vi "VFD Control Loop.vi"(8 "error in (no error)":errorcluster, 10 "VFD Notifier":refnum<notifier>, 11 "Message Queues":T2) -> (0 "error out":errorcluster)   [LabVIEW 2026]
uses:
  support/Message Queue/All Message Queues.ctl
  support/Message Queue/Message Cluster.ctl
  controls/VFD Notifier ctl.ctl
  Acquisition/Hardware Configuration.ctl
  controls/Durability Test Conditions.ctl
  Acquisition/Acquisition State.ctl
  VFD-Library-main/VFD-Library-main/Public/Action/Direction Selection.ctl
  support/Message Queue/Enqueue Message (Single).vi
  <vilib>/Utility/error.llb/Error Cluster From Error Code.vi
  <vilib>/ErrorRing/Error Ring.xnode
  Acquisition/Acquisition.lvlib
  support/Message Queue/Message Queue.lvlib
  VFD-Library-main/VFD-Library-main/VFD Library.lvlib
panel:
  in  "Cluster":T1={"Voltage"=0.0, "Current"=0.0, "Motor Speed"=0.0, "Fault"=TRUE, "Fault Messages"=[]}
  out "Faults":string[](array[string])
  out "Fault":bool
  out "Motor feedback\nspeed":dbl format="%#_13g"
  out "Current":dbl format="%#_13g"
  out "Voltage":dbl format="%#_13g"
  in  "IP Address":string="172.20.0.115"
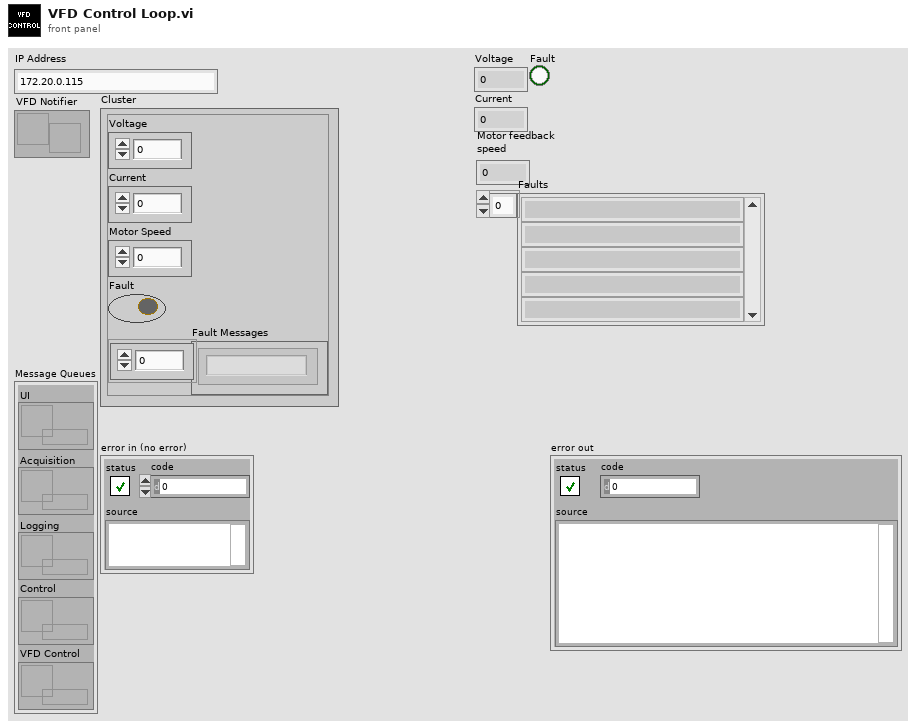
[diagram p1: front panel]
types:
  T1 = typedef "VFD Notifier ctl.ctl" = cluster{"Voltage":dbl, "Current":dbl, "Motor Speed":dbl, "Fault":bool, "Fault Messages":string[]}
  T2 = typedef "Message Queue.lvlib/All Message Queues.ctl" = cluster{"UI":refnum<queue>, "Acquisition":refnum<queue>, "Logging":refnum<queue>, "Control":refnum<queue>, "VFD Control":refnum<queue>}
  T3 = typedef "Acquisition.lvlib/Hardware Configuration.ctl" = cluster{"Analog Out array":dbl[], "Initialize Flag":bool, "Saftey Table Display":refnum<vi>, "Torque&Force":waveform(dbl)[][], "Calibration Data":waveform(dbl)[], "2D":dbl[][], "Analog In Task":refnum<k21>, "Digital In Task":refnum<k21>, "Analog Out Task":refnum<k21>, "Digital Out Task":refnum<k21>, "Digital Out Array":bool[], "Current Cycle Count":refnum<vi>, "Cycle Count":u64, "Headers":string[], "Sweep Interval":u64, "Delay":u64, "TestConfigDisplay":refnum<vi>, "50psi Conversion":dbl[], "1245N15 Conversion":dbl[], "MX06F Conversion":dbl[], "# of Test Cycles":u64, "60psi Conversion":dbl[], "100psi Conversion":dbl[], "200psi Conversion":dbl[], "1000psi Conversion":dbl[], "2000psi Conversion":dbl[], "5000psi Conversion":dbl[], "MX09F Conversion":dbl[], "MX19F Conversion":dbl[], "DUT VALVE POSITION":refnum<vi>, "INTAKE VALVE POSITION":refnum<vi>, "Table Control":refnum<vi>, "Table Control":string[][], "Max Vacuum":dbl, "RPM Ramp Ref":refnum<vi>, "Free Air Flow Ref":refnum<vi>, "Press Stable Ref":refnum<vi>, "Press Decay Ref":refnum<vi>, "Pulley Ratio":dbl, "Calculated Pulley Ratio":refnum<vi>, "Durability Test Conditions":T4, "# of Durab Steps":dbl, "manual aquire timer":dbl, "Durability Test Conditions Initial":T4}
  T4 = typedef "Durability Test Conditions.ctl" = cluster{"Step #s":dbl[], "RPMs":dbl[], "Step Durations":dbl[], "Step Delays":dbl[], "Test Cycles":dbl}
  T5 = typedef "Acquisition.lvlib/Acquisition State.ctl" = enum16{"Idle", "Acquiring"}
  T6 = typedef "VFD Library.lvlib/Direction Selection.ctl" = u16
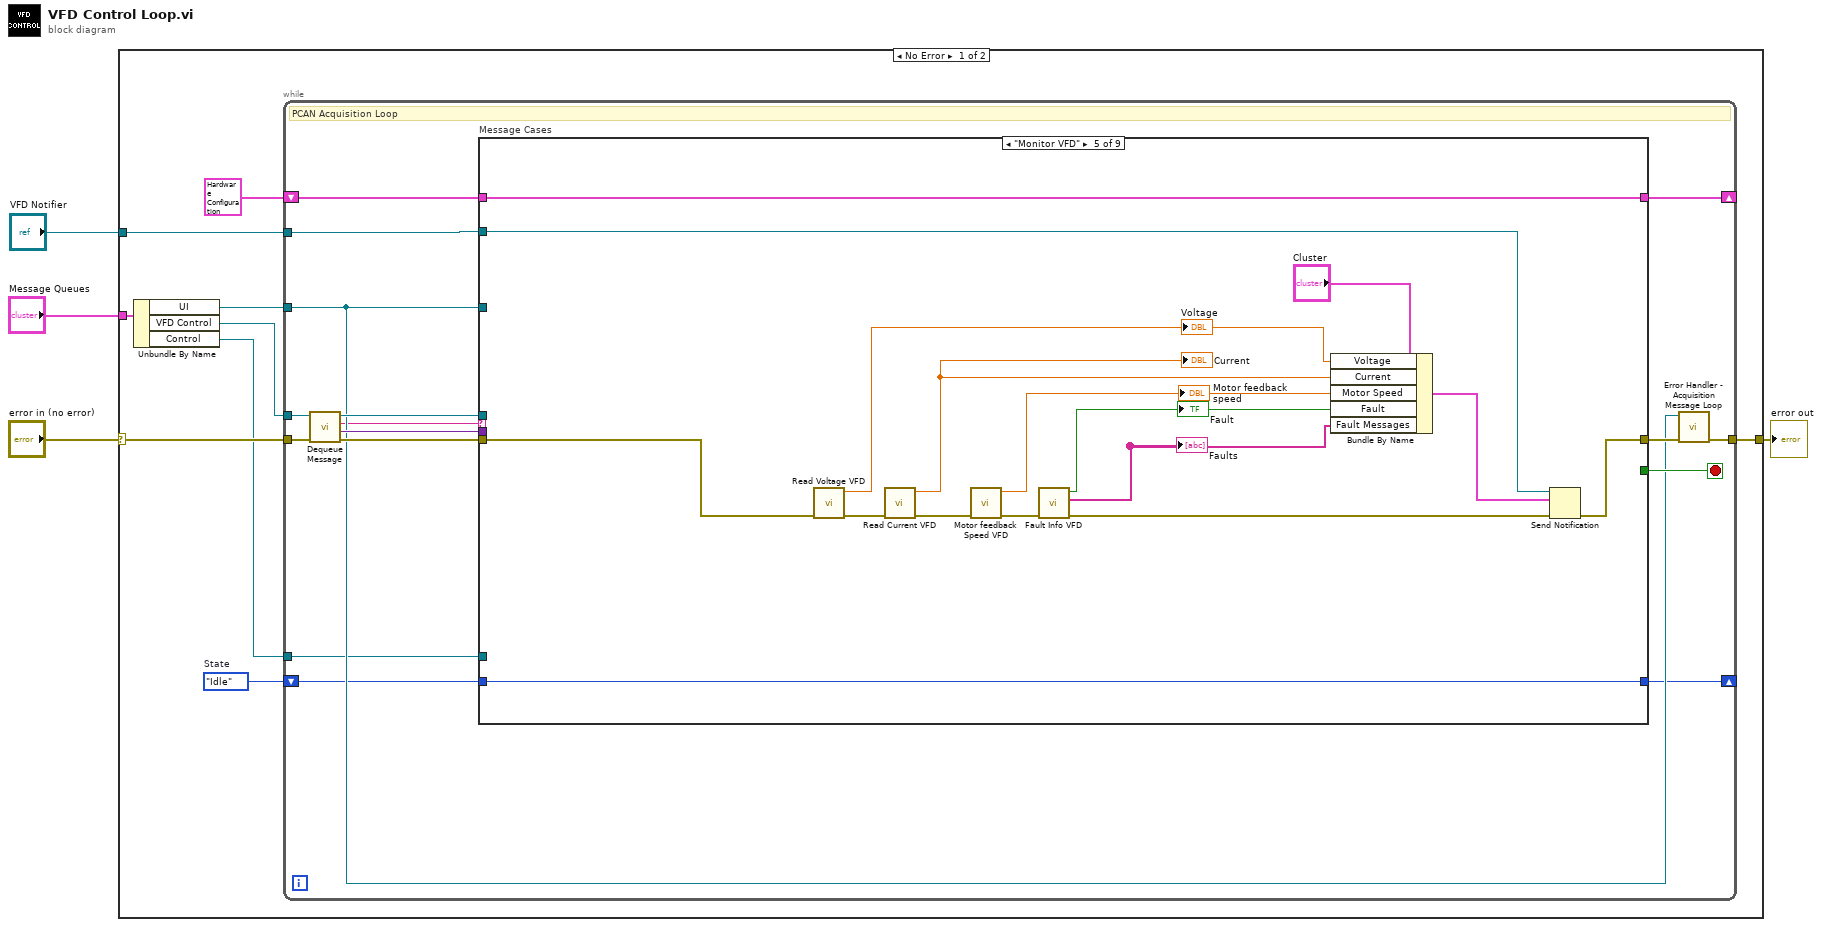
[diagram p0: block diagram]
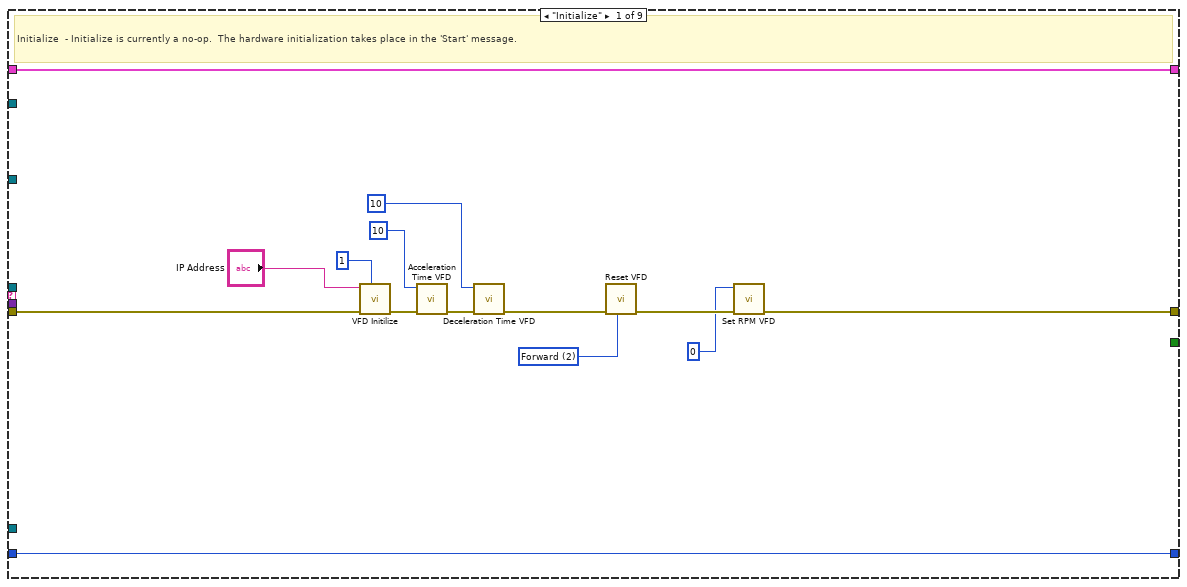
[diagram p2: hidden frame]
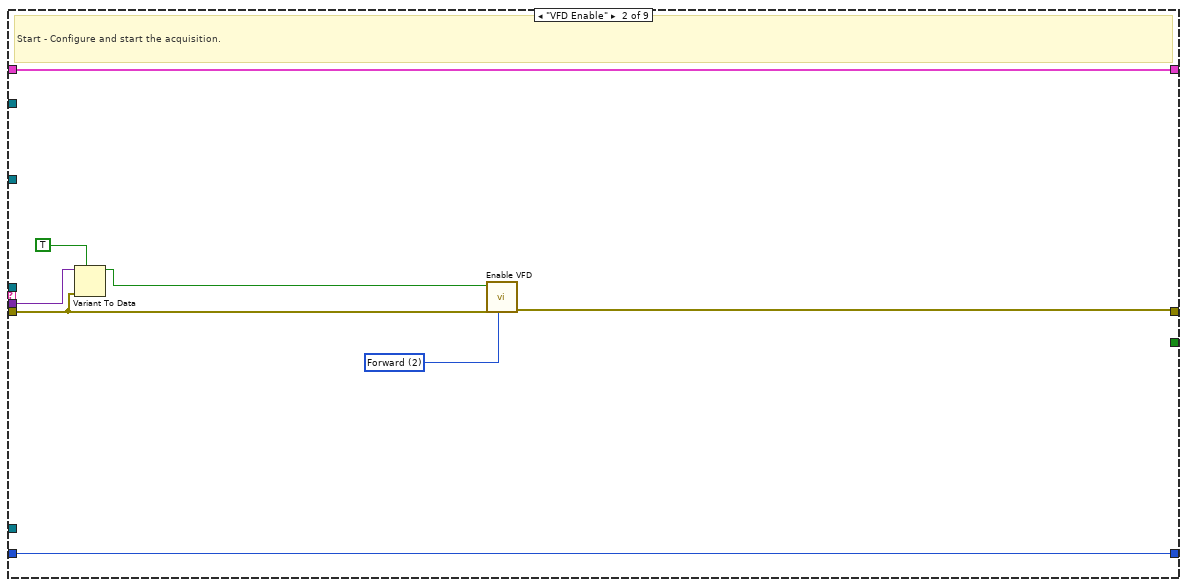
[diagram p3: hidden frame]
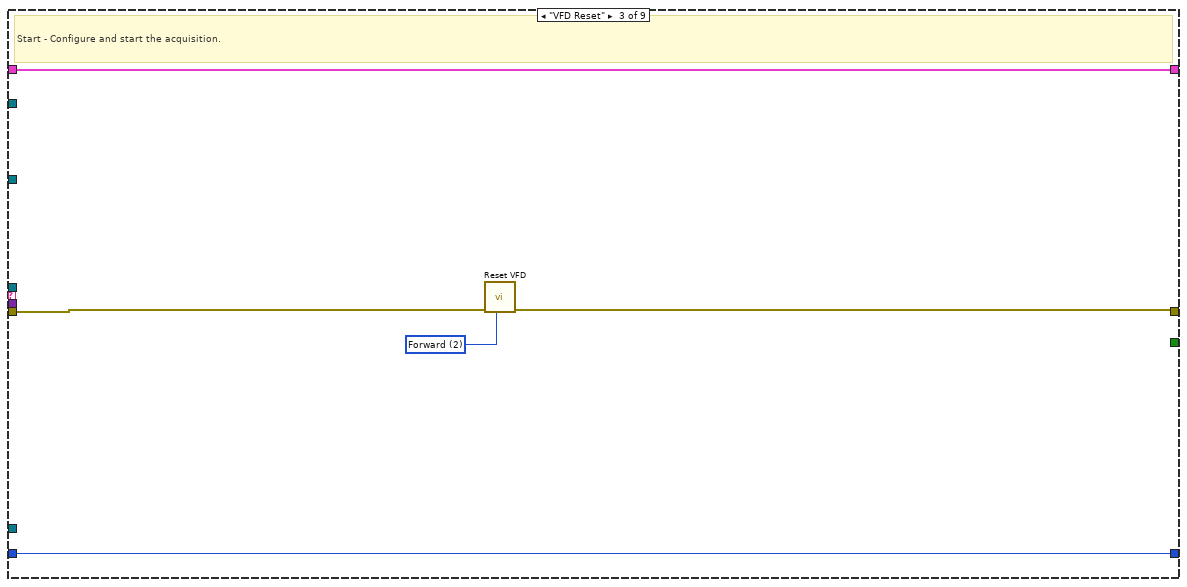
[diagram p4: hidden frame]
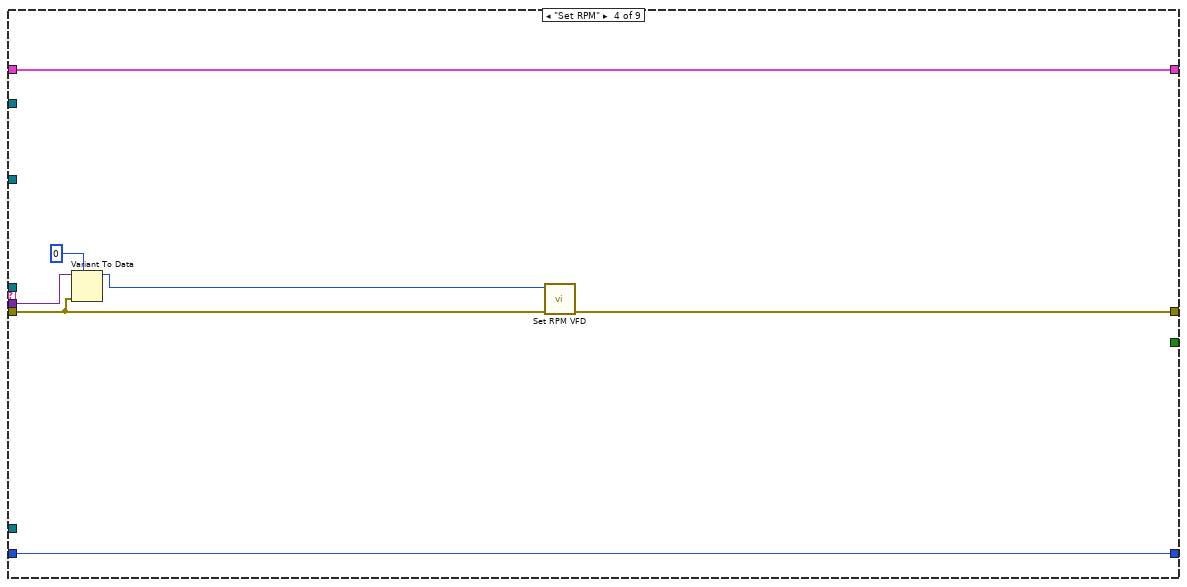
[diagram p5: hidden frame]
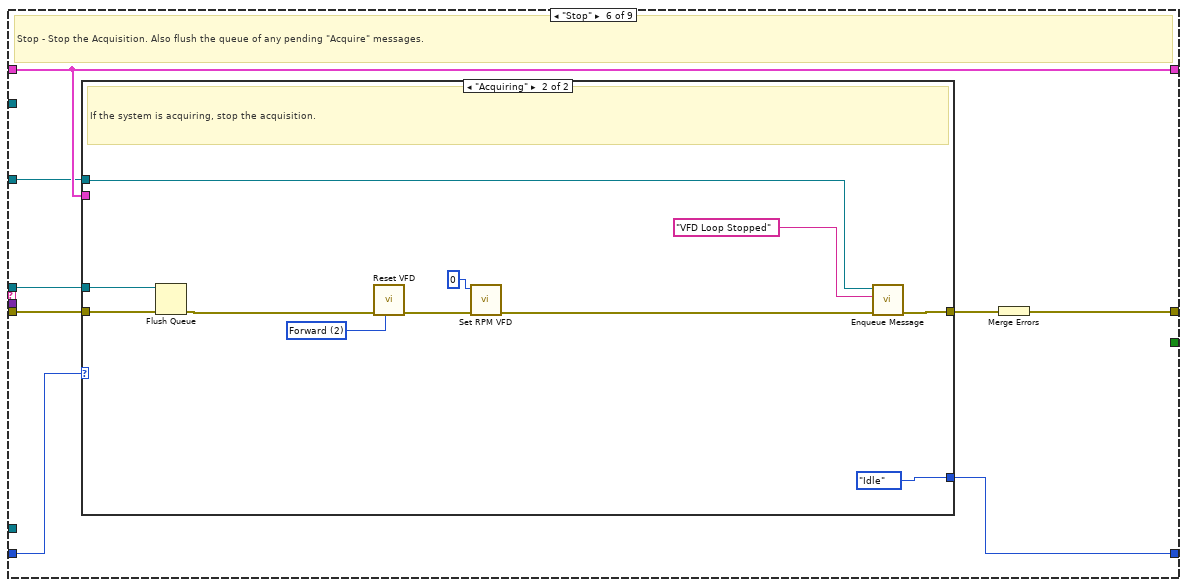
[diagram p6: hidden frame]
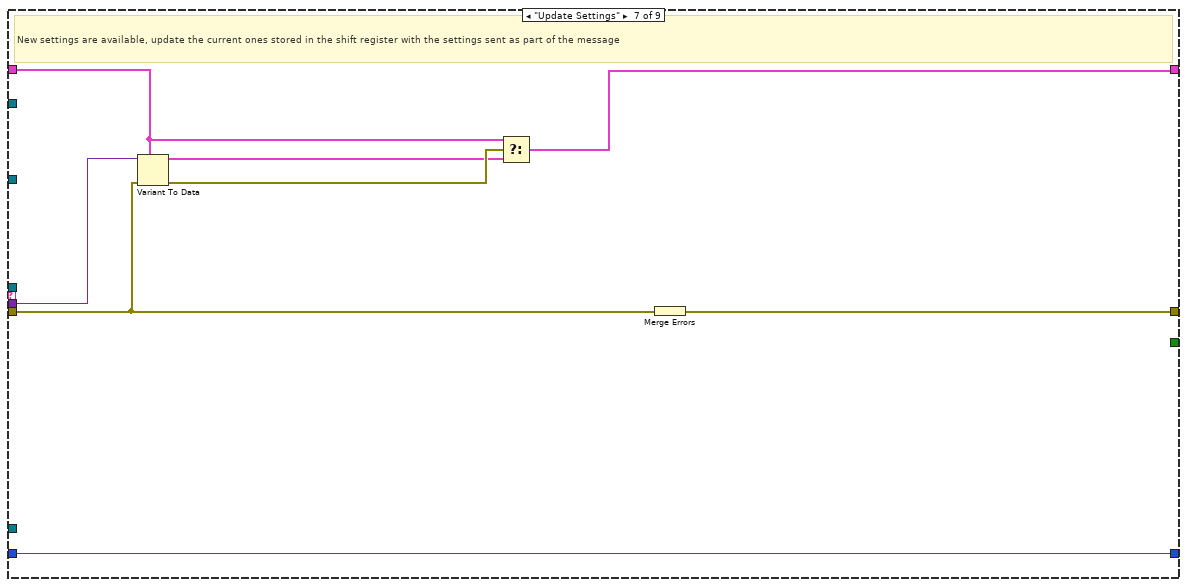
[diagram p8: hidden frame]
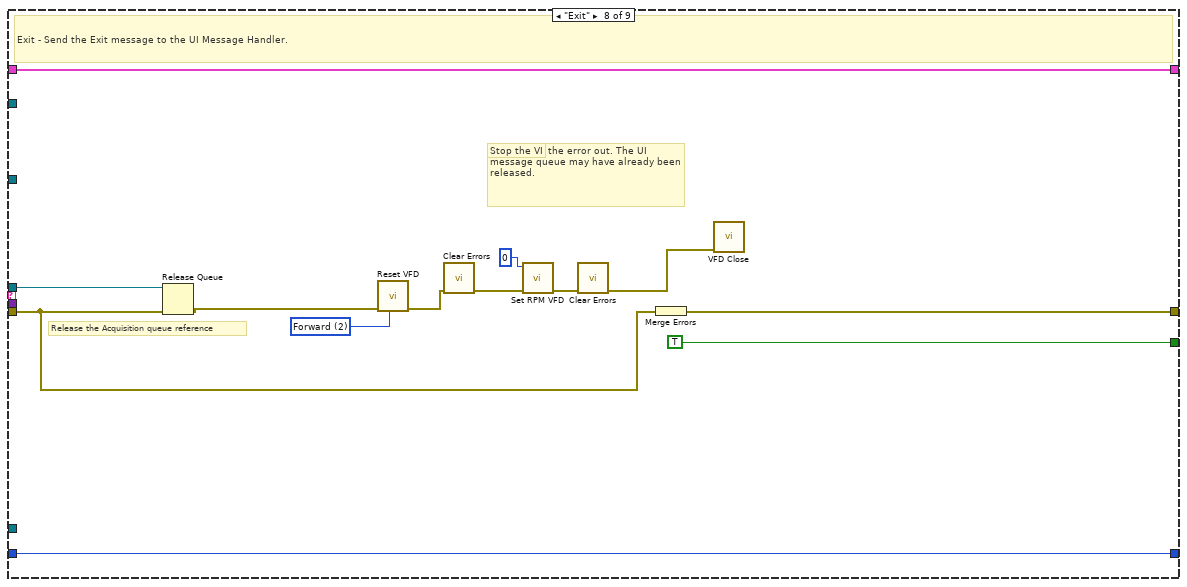
[diagram p9: hidden frame]
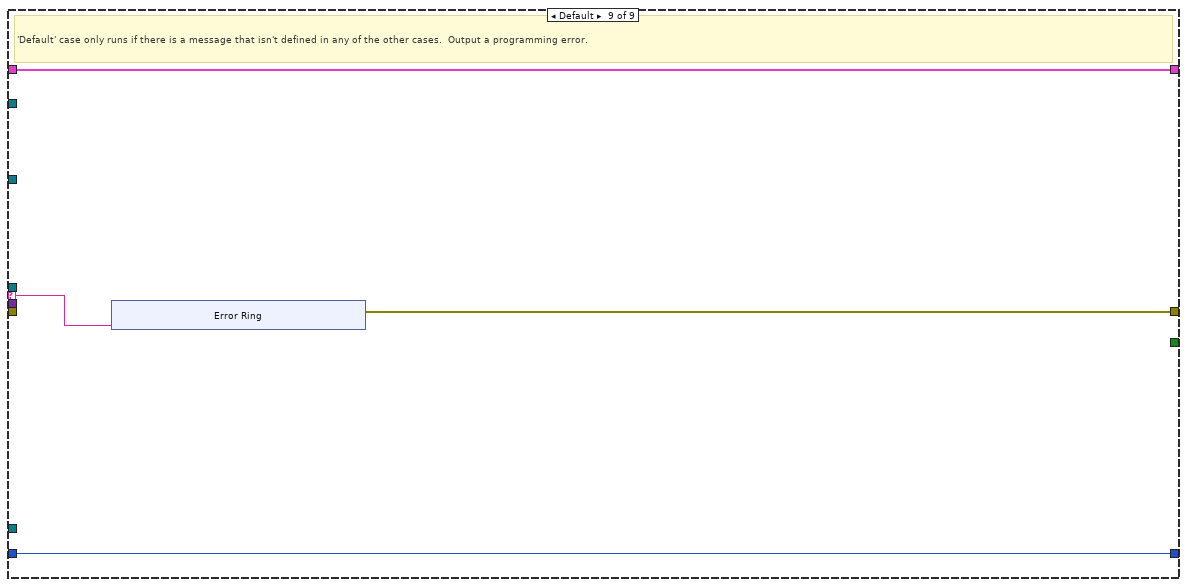
[diagram p10: hidden frame]
diagram:
  n1 = case shown="No Error" "error in (no error)" {
    selector: "error in (no error)" -> [w10 w133]
    tunnel: "Message Queues" -> [w13 _]
    tunnel: [w12 w133] -> w3
    tunnel: "VFD Notifier" -> [w5 _]
    frame No Error {
      w8 = Acquisition_State."Idle"  # State
      n2 = Unbundle By Name(w13) -> ("UI"=w9:refnum<queue>, "VFD Control"=w6:refnum<queue>, "Control"=w7:refnum<queue>)
      n3 = while {
        tunnel: w6 -> [w22]
        shift-right: [w28] -> _
        shift-left: T3 {"Analog Out array"=[], "Initialize Flag"=FALSE, "Saftey Table Display"=refnum, "Torque&Force"=[], "Calibration Data"=[], "2D"=[], "Analog In Task"="", "Digital In Task"="", "Analog Out Task"="", "Digital Out Task"="", "Digital Out Array"=[], "Current Cycle Count"=refnum, "Cycle Count"=0, "Headers"=[], "Sweep Interval"=0, "Delay"=0, "TestConfigDisplay"=refnum, "50psi Conversion"=[], "1245N15 Conversion"=[], "MX06F Conversion"=[], "# of Test Cycles"=0, "60psi Conversion"=[], "100psi Conversion"=[], "200psi Conversion"=[], "1000psi Conversion"=[], "2000psi Conversion"=[], "5000psi Conversion"=[], "MX09F Conversion"=[], "MX19F Conversion"=[], "DUT VALVE POSITION"=refnum, "INTAKE VALVE POSITION"=refnum, "Table Control"=refnum, "Table Control"=[], "Max Vacuum"=0.0, "RPM Ramp Ref"=refnum, "Free Air Flow Ref"=refnum, "Press Stable Ref"=refnum, "Press Decay Ref"=refnum, "Pulley Ratio"=0.0, "Calculated Pulley Ratio"=refnum, "Durability Test Conditions"={"Step #s"=[], "RPMs"=[], "Step Durations"=[], "Step Delays"=[], "Test Cycles"=0.0}, "# of Durab Steps"=0.0, "manual aquire timer"=0.0, "Durability Test Conditions Initial"={"Step #s"=[], "RPMs"=[], "Step Durations"=[], "Step Delays"=[], "Test Cycles"=0.0}} ("Data Cluster") -> [w29]
        tunnel: w9 -> [w19]
        shift-right: [w17] -> _
        shift-left: w8 -> [w18]
        tunnel: w7 -> [w16]
        tunnel: w10 -> [w26]
        tunnel: [w20] -> w12
        tunnel: w5 -> [w15]
        stop <- w27 stop-if-true
        # "PCAN Acquisition Loop"
        n4 = call "Dequeue Message.vi"("error in (no error)"=w26, "Message Queue"=w22) -> ("error out"=w25:errorcluster, "Message Data"=w24:variant, "Message"=w14:string, "dup Message Queue"=w23:refnum<queue>)  [unwired: 6 in]
        n5 = case "Message Cases" shown="\"Monitor VFD\"" w14 {
          selector: w14 -> [_ _ _ _ _ _ _ _ w124]
          tunnel: w23 -> [_ _ _ _ _ w84 _ w119 _]
          tunnel: w25 -> [w35 w47 w54 w60 w75 w86 w102 w116 _]
          tunnel: [w32 w49 w53 w61 w72 w87 w108 w120 w123] -> w21
          tunnel: w29 -> [w42 w50 w55 w62 w79 w85 w104 w117 w125]
          tunnel: [w42 w50 w55 w62 w79 w85 w103 w117 w125] -> w28
          tunnel: [_ _ _ _ _ _ _ TRUE _] -> w27
          tunnel: w24 -> [_ w46 _ w59 _ _ w107 _ _]
          tunnel: w19 -> [_ _ _ _ _ w83 _ _ _]
          tunnel: w18 -> [w43 w51 w56 w63 w74 w82 w101 w118 w122]
          tunnel: [w43 w51 w56 w63 w74 w81 w101 w118 w122] -> w17
          tunnel: w16 -> [_ _ _ _ _ _ _ _ _]
          tunnel: w15 -> [_ _ _ _ w71 _ _ _ _]
          frame "Initialize" {
            w31 = T6 2 items=["Reverse"=0, "Forward"=2] ("Direction")
            # "Initialize  - Initialize is currently a no-op.  The hardware initialization takes place in the 'Start' message."
            n6 = call "VFD Initilize.vi"("Slave ID (255)"=u8 1, "error In"=w35, "IP Address"="IP Address") -> ("error out"=w40:errorcluster)  [unwired: 8 in]
            n7 = call "Acceleration Time VFD.vi"("error In"=w40, "Set Acceleration time"=u16 10) -> ("error out"=w39:errorcluster)  [unwired: 9 in]
            n8 = call "Deceleration Time VFD.vi"("error In"=w39, "Set Deceleration time"=u16 10) -> ("error out"=w34:errorcluster)  [unwired: 9 in]
            n9 = call "Reset VFD.vi"("Direction"=w31, "error In"=w34) -> ("error out"=w33:errorcluster)  [unwired: 9 in]
            n10 = call "Set RPM VFD.vi"("error In"=w33, "Set RPM"=u16 0) -> ("error out"=w32:errorcluster)  [unwired: 9 in]
          }
          frame "VFD Enable" {
            w48 = T6 2 items=["Reverse"=0, "Forward"=2] ("Direction")
            # "Start - Configure and start the acquisition."
            n11 = Variant To Data(error in=w47, type=TRUE, Variant=w46) -> (data=w44:bool)  [unwired: 1 out]
            n12 = call "Enable VFD.vi"("Direction"=w48, "error In"=w47, "Enable"=w44) -> ("error out"=w49:errorcluster)  [unwired: 8 in]
          }
          frame "VFD Reset" {
            w52 = T6 2 items=["Reverse"=0, "Forward"=2] ("Direction")
            # "Start - Configure and start the acquisition."
            n13 = call "Reset VFD.vi"("Direction"=w52, "error In"=w54) -> ("error out"=w53:errorcluster)  [unwired: 9 in]
          }
          frame "Set RPM" {
            n14 = Variant To Data(error in=w60, type=u16 0 ("Set RPM"), Variant=w59) -> (data=w57:u16)  [unwired: 1 out]
            n15 = call "Set RPM VFD.vi"("error In"=w60, "Set RPM"=w57) -> ("error out"=w61:errorcluster)  [unwired: 9 in]
          }
          frame "Monitor VFD" {
            n16 = call "Read Voltage VFD.vi"("error In"=w75) -> ("error out"=w78:errorcluster, "Voltage"=w66:dbl)  [unwired: 9 in]
            "Voltage" <- w66
            n17 = call "Read Current VFD.vi"("error In"=w78) -> ("error out"=w77:errorcluster, "Current"=w67:dbl)  [unwired: 9 in]
            "Current" <- w67
            n18 = call "Motor feedback Speed VFD.vi"("error In"=w77) -> ("error out"=w76:errorcluster, "Motor feedback\nspeed"=w68:dbl)  [unwired: 9 in]
            "Motor feedback\nspeed" <- w68
            n19 = call "Fault Info VFD.vi"("error In"=w76) -> ("error out"=w73:errorcluster, "Faults"=w70:string[], "Fault"=w69:bool)  [unwired: 8 in]
            "Fault" <- w69
            "Faults" <- w70
            n20 = Bundle By Name(cluster="Cluster", "Voltage"=w66, "Current"=w67, "Motor Speed"=w68, "Fault"=w69, "Fault Messages"=w70) -> (w64:T1)
            n21 = Send Notification(notification=w64, notifier=w71, error in (no error)=w73) -> (error out=w72:errorcluster)  [unwired: 1 out]
          }
          frame "Stop" {
            # "Stop - Stop the Acquisition. Also flush the queue of any pending \"Acquire\" messages."
            n22 = case shown="\"Acquiring\"" w82 {
              selector: w82 -> [w89 _]
              tunnel: w86 -> [w88 w100]
              tunnel: w85 -> [_ _]
              tunnel: w84 -> [_ w99]
              tunnel: w83 -> [_ w98]
              tunnel: [w89 Acquisition_State."Idle" ("State")] -> w81
              tunnel: [w88 w97] -> w80
              frame "Idle", Default {
                # "The system is already idle. Ignore the \"Stop\" message."
              }
              frame "Acquiring" {
                w94 = T6 2 items=["Reverse"=0, "Forward"=2] ("Direction")
                # "If the system is acquiring, stop the acquisition."
                n23 = Flush Queue(queue=w99, error in (no error)=w100) -> (error out=w91:errorcluster)  [unwired: 2 out]
                n24 = call "Reset VFD.vi"("Direction"=w94, "error In"=w91) -> ("error out"=w93:errorcluster)  [unwired: 9 in]
                n25 = call "Set RPM VFD.vi"("error In"=w93, "Set RPM"=u16 0) -> ("error out"=w90:errorcluster)  [unwired: 9 in]
                n26 = call-poly "Enqueue Message.vi"("error in (no error)"=w90, "Message"="VFD Loop Stopped", "Message Queue"=w98) -> ("error out"=w97:errorcluster)  [unwired: 7 in, 1 out]
              }
            }
            n27 = Merge Errors(w80) -> (w87:errorcluster)
          }
          frame "Update Settings" {
            # "New settings are available, update the current ones stored in the shift register with the settings sent as part of the message"
            n28 = Variant To Data(error in=w102, type=w104, Variant=w107) -> (data=w105:T3, error out=w106:errorcluster)
            n29 = Select(t=w104, s=w106, f=w105) -> (s? t:f=w103:T3)
            n30 = Merge Errors(w102) -> (w108:errorcluster)
          }
          frame "Exit" {
            w115 = T6 2 items=["Reverse"=0, "Forward"=2] ("Direction")
            # "Don't check the error out. The UI message queue may have already been released."
            # "Release the Acquisition queue reference"
            # "Stop the VI"
            # "Exit - Send the Exit message to the UI Message Handler."
            n31 = Release Queue(queue=w119, error in (no error)=w116) -> (error out=w113:errorcluster)  [unwired: 1 in, 2 out]
            n32 = call "Reset VFD.vi"("Direction"=w115, "error In"=w113) -> ("error out"=w112:errorcluster)  [unwired: 9 in]
            n33 = call <vilib>:"Clear Errors.vi"("error in (no error)"=w112) -> ("error out"=w111:errorcluster)  [unwired: 5 in, 1 out]
            n34 = call "Set RPM VFD.vi"("error In"=w111, "Set RPM"=u16 0) -> ("error out"=w110:errorcluster)  [unwired: 9 in]
            n35 = call <vilib>:"Clear Errors.vi"("error in (no error)"=w110) -> ("error out"=w109:errorcluster)  [unwired: 5 in, 1 out]
            n36 = Merge Errors(w116) -> (w120:errorcluster)
            n37 = call "VFD Close.vi"("error In"=w109) -> ()  [unwired: 10 in, 1 out]
          }
          frame Default {
            # "'Default' case only runs if there is a message that isn't defined in any of the other cases.  Output a programming error."
            n38 = xnode "Error Ring"("parameter 0"=w124) -> ("error out"=w123:errorcluster)
          }
        }
        n39 = call "Error Handler - Acquisition Message Loop.vi"("error in (no error)"=w21, "Message Queue"=w19) -> ("dup error in"=w20:errorcluster)  [unwired: 8 in, 1 out]
      }
    }
    frame Error {
    }
  }
  "error out" <- w3
